vi "cm2nm_create_graph_of_session.vi"(1 "CollectionOfSpots":T1[](array[typedef])) -> (0 "X/Y plot array of spots":cluster{dbl[], dbl[]}[](array[cluster]))   [LabVIEW 2011]
uses:
  cm2nm_coordinate_information_v2.ctl
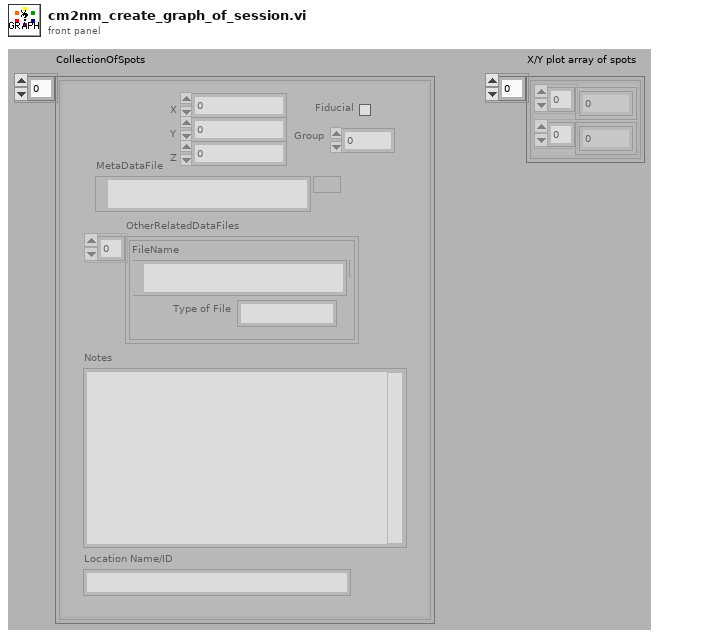
[diagram p1: front panel]
types:
  T1 = typedef "cm2nm_coordinate_information_v2.ctl" = cluster{"MetaDataFile":path, "X":dbl, "Y":dbl, "Z":dbl, "Group":i32, "Rotation":dbl[unit], "Fiducial":bool, "Magnification":dbl, "Working_Distance":dbl, "Notes":string, "Location Name/ID":string, "OtherRelatedDataFiles":cluster{"Type of File":string, "FileName":path}[], "Available":bool}
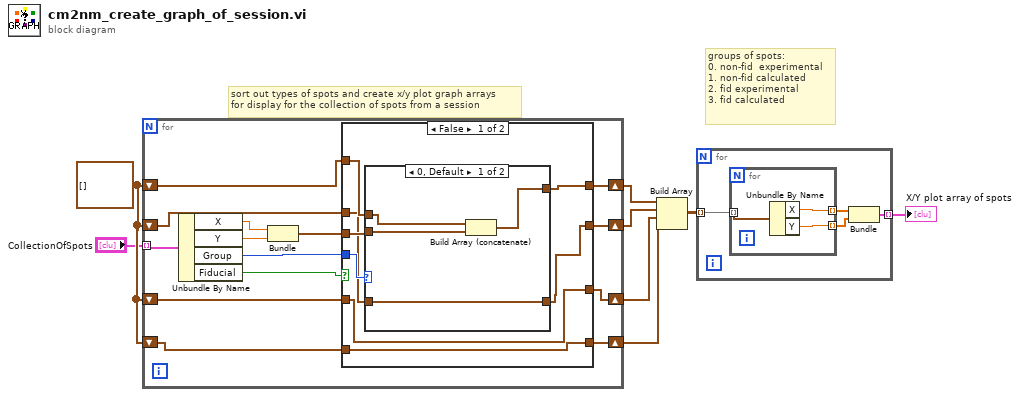
[diagram p0: block diagram]
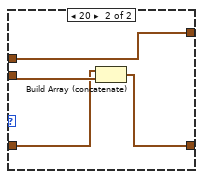
[diagram p2: hidden frame]
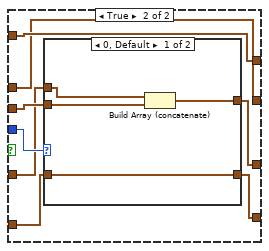
[diagram p3: hidden frame]
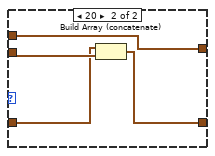
[diagram p4: hidden frame]
diagram:
  w8 = cluster{"X":dbl, "Y":dbl}[] []
  # "groups of spots:\n0. non-fid  experimental\n1. non-fid calculated\n2. fid experimental\n3. fid calculated"
  # "sort out types of spots and create x/y plot graph arrays \nfor display for the collection of spots from a session"
  n1 = for {
    tunnel: "CollectionOfSpots" -> [w22] mode=indexing
    shift-right: [w16] -> w3
    shift-left: w8 -> [w15]
    shift-right: [w14] -> w4
    shift-left: w8 -> [w13]
    shift-right: [w12] -> w5
    shift-left: w8 -> [w11]
    shift-right: [w10] -> w2
    shift-left: w8 -> [w9]
    n2 = Unbundle By Name(w22) -> ("X"=w20:dbl, "Y"=w21:dbl, "Group"=w18:i32, "Fiducial"=w19:bool)
    n3 = Bundle("X"=w20, "Y"=w21) -> (w17:cluster{"X":dbl, "Y":dbl})  [unwired: 1 in]
    n4 = case shown="False" w19 {
      tunnel: w18 -> [w27 w46]
      tunnel: w17 -> [w30 w45]
      tunnel: [w25 w39] -> w16
      tunnel: w15 -> [w24 w39]
      tunnel: [w26 w43] -> w14
      tunnel: w13 -> [w26 w42]
      tunnel: [w23 w41] -> w12
      tunnel: w11 -> [w23 w40]
      tunnel: [w29 w44] -> w10
      tunnel: w9 -> [w28 w44]
      frame False {
        n5 = case shown="0, Default" w27 {
          tunnel: w30 -> [w34 w37]
          tunnel: [w33 w35] -> w29
          tunnel: w28 -> [w32 w35]
          tunnel: [w31 w38] -> w25
          tunnel: w24 -> [w31 w36]
          frame 0, Default {
            n6 = Build Array (concatenate)(w32, w34) -> (w33:cluster{"X":dbl, "Y":dbl}[])
          }
          frame 20 {
            n7 = Build Array (concatenate)(w36, w37) -> (w38:cluster{"X":dbl, "Y":dbl}[])
          }
        }
      }
      frame True {
        n8 = case shown="0, Default" w46 {
          tunnel: w45 -> [w50 w53]
          tunnel: [w49 w51] -> w43
          tunnel: w42 -> [w48 w51]
          tunnel: [w47 w54] -> w41
          tunnel: w40 -> [w47 w52]
          frame 0, Default {
            n9 = Build Array (concatenate)(w48, w50) -> (w49:cluster{"X":dbl, "Y":dbl}[])
          }
          frame 20 {
            n10 = Build Array (concatenate)(w52, w53) -> (w54:cluster{"X":dbl, "Y":dbl}[])
          }
        }
      }
    }
  }
  n11 = Build Array(w2, w3, w4, w5) -> (w6:cluster{"X":dbl, "Y":dbl}[][])
  n12 = for {
    tunnel: w6 -> [w58] mode=indexing
    tunnel: [w55] -> w7 mode=indexing
    n13 = for {
      tunnel: w58 -> [w61] mode=indexing
      tunnel: [w60] -> w56 mode=indexing
      tunnel: [w59] -> w57 mode=indexing
      n14 = Unbundle By Name(w61) -> ("X"=w60:dbl, "Y"=w59:dbl)
    }
    n15 = Bundle(w56, w57) -> (w55:cluster{dbl[], dbl[]})  [unwired: 1 in]
  }
  "X/Y plot array of spots" <- w7
